vi "TCPR.vi"(0 "connection ID":refnum<k5>, 2 "错误输入（无错误）":errorcluster) -> (1 "吸液阀状态":i32, 3 "内部压力":dbl format="%.3f", 4 "外部压力":dbl format="%#.3f", 5 "连接ID输出":refnum<k5>, 6 "跟踪压力":dbl format="%.3f", 7 "错误输出":errorcluster, 8 "当前泵容量":dbl format="%.3f", 9 "排液阀状态":i32)   [LabVIEW 2014]
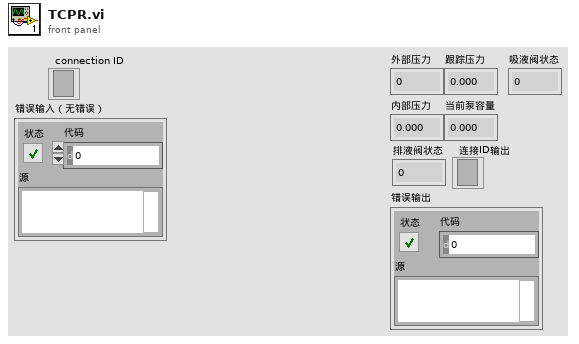
[diagram p1: front panel]
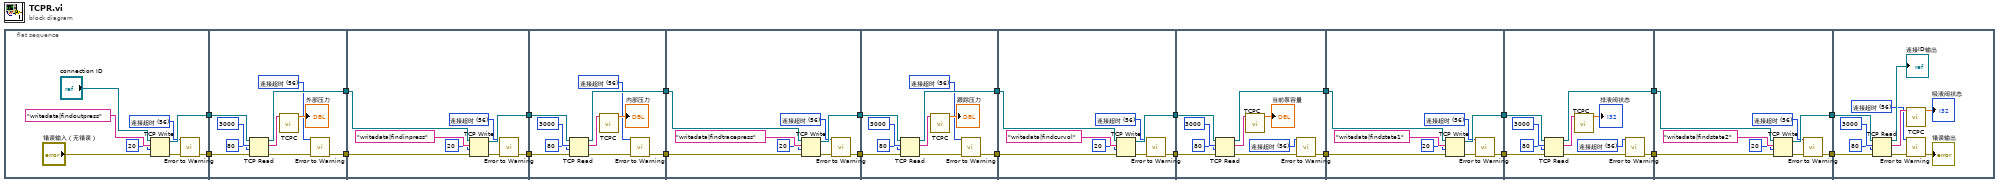
[diagram p0: block diagram]
diagram:
  n1 = flat-sequence {
    tunnel: [w24] -> w22
    tunnel: [w28] -> w21
    tunnel: w22 -> [w40]
    tunnel: w21 -> [w39]
    tunnel: [w36] -> w20
    tunnel: [w34] -> w5
    tunnel: w20 -> [w48]
    tunnel: [w46] -> w19
    tunnel: [w41] -> w6
    tunnel: w5 -> [w45]
    tunnel: w19 -> [w58]
    tunnel: [w55] -> w18
    tunnel: w6 -> [w54]
    tunnel: [w52] -> w4
    tunnel: w18 -> [w66]
    tunnel: [w64] -> w17
    tunnel: [w59] -> w7
    tunnel: w4 -> [w63]
    tunnel: w17 -> [w76]
    tunnel: [w73] -> w16
    tunnel: w7 -> [w72]
    tunnel: [w70] -> w3
    tunnel: w16 -> [w84]
    tunnel: [w82] -> w15
    tunnel: [w78] -> w8
    tunnel: w3 -> [w81]
    tunnel: w15 -> [w94]
    tunnel: [w91] -> w14
    tunnel: w8 -> [w90]
    tunnel: [w88] -> w2
    tunnel: w14 -> [w102]
    tunnel: [w100] -> w13
    tunnel: [w97] -> w9
    tunnel: w2 -> [w99]
    tunnel: w13 -> [w112]
    tunnel: [w109] -> w12
    tunnel: w9 -> [w108]
    tunnel: [w106] -> w1
    tunnel: w12 -> [w120]
    tunnel: [w118] -> w11
    tunnel: [w115] -> w10
    tunnel: w1 -> [w117]
    tunnel: w11 -> [w130]
    tunnel: w10 -> [w126]
    frame #0 {
      w23 = 56 items=["无错误", "参数错误", "内存已满", "超出区域", "文件结束", "文件已打开", "一般文件IO错误", "未找到文件", "文件权限错误", "磁盘已满", "路径副本", "打开过多文件", "未启用", "未找到资源文件", "无法添加资源", "未找到资源", "未找到图像", "图像内存错误", "画笔不存在", "配置错误类型", "配置未找到解析段", "配置解析错误", "配置内存错误", "错误外部代码格式", "错误外部代码偏移量", "外部代码不存在", "空窗口", "销毁窗口错误", "空菜单", "打印已中止", "错误打印记录", "打印驱动程序错误", "打印时窗口错误", "打印时内存错误", "打印对话框错误", "一般打印错误", "无效设备引用句柄", "设备未找到", "设备参数错误", "设备单位错误", "无法打开设备", "设备调用已中止", "一般错误", "用户已取消", "对象ID过低", "对象ID过高", "对象不在堆中", "未知的堆", "错误DefProc ID", "DefProc不在表格中", "范围外信息", "空方法", "未知信息", "不支持管理器调用", "错误地址", "连接过程中", "连接超时", "连接过程中", "不支持网络属性", "网络错误", "正在使用的地址", "系统缺少内存", "连接已中止", "连接已拒绝", "连接未建立", "连接已建立", "连接已关闭", "初始化错误（交互应用程序管理器）", "错误事件发生", "等待无约束事件发生处理程序", "事件发生队列溢出", "错误路径", "未发出信号量", "未识别类型（交互应用程序管理器）"] ("1st Error to Convert")
      n2 = TCP Write(connection ID="connection ID", data in="writedata|findoutpress" ("数据输入"), error in (no error)="错误输入（无错误）", 9:20 ("超时毫秒(25000)")) -> (connection ID out=w28:refnum<k5>, error out=w25:errorcluster)  [unwired: 1 out]
      n3 = call <vilib>:"Error to Warning.vi"("1st Error to Convert"=w23, "error in"=w25) -> ("warning out"=w24:errorcluster)  [unwired: 13 in]
    }
    frame #1 {
      w31 = 56 items=["无错误", "参数错误", "内存已满", "超出区域", "文件结束", "文件已打开", "一般文件IO错误", "未找到文件", "文件权限错误", "磁盘已满", "路径副本", "打开过多文件", "未启用", "未找到资源文件", "无法添加资源", "未找到资源", "未找到图像", "图像内存错误", "画笔不存在", "配置错误类型", "配置未找到解析段", "配置解析错误", "配置内存错误", "错误外部代码格式", "错误外部代码偏移量", "外部代码不存在", "空窗口", "销毁窗口错误", "空菜单", "打印已中止", "错误打印记录", "打印驱动程序错误", "打印时窗口错误", "打印时内存错误", "打印对话框错误", "一般打印错误", "无效设备引用句柄", "设备未找到", "设备参数错误", "设备单位错误", "无法打开设备", "设备调用已中止", "一般错误", "用户已取消", "对象ID过低", "对象ID过高", "对象不在堆中", "未知的堆", "错误DefProc ID", "DefProc不在表格中", "范围外信息", "空方法", "未知信息", "不支持管理器调用", "错误地址", "连接过程中", "连接超时", "连接过程中", "不支持网络属性", "网络错误", "正在使用的地址", "系统缺少内存", "连接已中止", "连接已拒绝", "连接未建立", "连接已建立", "连接已关闭", "初始化错误（交互应用程序管理器）", "错误事件发生", "等待无约束事件发生处理程序", "事件发生队列溢出", "错误路径", "未发出信号量", "未识别类型（交互应用程序管理器）"] ("1st Error to Convert")
      n4 = TCP Read(connection ID=w39, bytes to read=3000 ("读取的字节"), error in (no error)=w40, 9:80 ("超时毫秒(25000)")) -> (connection ID out=w36:refnum<k5>, data out=w38:string, error out=w35:errorcluster)  [unwired: 1 in]
      n5 = call "TCPC.vi"("data out"=w38) -> ("offset past number"=→"外部压力":dbl)  [unwired: 10 in]
      n6 = call <vilib>:"Error to Warning.vi"("1st Error to Convert"=w31, "error in"=w35) -> ("warning out"=w34:errorcluster)  [unwired: 13 in]
    }
    frame #2 {
      w42 = 56 items=["无错误", "参数错误", "内存已满", "超出区域", "文件结束", "文件已打开", "一般文件IO错误", "未找到文件", "文件权限错误", "磁盘已满", "路径副本", "打开过多文件", "未启用", "未找到资源文件", "无法添加资源", "未找到资源", "未找到图像", "图像内存错误", "画笔不存在", "配置错误类型", "配置未找到解析段", "配置解析错误", "配置内存错误", "错误外部代码格式", "错误外部代码偏移量", "外部代码不存在", "空窗口", "销毁窗口错误", "空菜单", "打印已中止", "错误打印记录", "打印驱动程序错误", "打印时窗口错误", "打印时内存错误", "打印对话框错误", "一般打印错误", "无效设备引用句柄", "设备未找到", "设备参数错误", "设备单位错误", "无法打开设备", "设备调用已中止", "一般错误", "用户已取消", "对象ID过低", "对象ID过高", "对象不在堆中", "未知的堆", "错误DefProc ID", "DefProc不在表格中", "范围外信息", "空方法", "未知信息", "不支持管理器调用", "错误地址", "连接过程中", "连接超时", "连接过程中", "不支持网络属性", "网络错误", "正在使用的地址", "系统缺少内存", "连接已中止", "连接已拒绝", "连接未建立", "连接已建立", "连接已关闭", "初始化错误（交互应用程序管理器）", "错误事件发生", "等待无约束事件发生处理程序", "事件发生队列溢出", "错误路径", "未发出信号量", "未识别类型（交互应用程序管理器）"] ("1st Error to Convert")
      n7 = TCP Write(connection ID=w48, data in="writedata|findinpress" ("数据输入"), error in (no error)=w45, 9:20 ("超时毫秒(25000)")) -> (connection ID out=w46:refnum<k5>, error out=w43:errorcluster)  [unwired: 1 out]
      n8 = call <vilib>:"Error to Warning.vi"("1st Error to Convert"=w42, "error in"=w43) -> ("warning out"=w41:errorcluster)  [unwired: 13 in]
    }
    frame #3 {
      w49 = 56 items=["无错误", "参数错误", "内存已满", "超出区域", "文件结束", "文件已打开", "一般文件IO错误", "未找到文件", "文件权限错误", "磁盘已满", "路径副本", "打开过多文件", "未启用", "未找到资源文件", "无法添加资源", "未找到资源", "未找到图像", "图像内存错误", "画笔不存在", "配置错误类型", "配置未找到解析段", "配置解析错误", "配置内存错误", "错误外部代码格式", "错误外部代码偏移量", "外部代码不存在", "空窗口", "销毁窗口错误", "空菜单", "打印已中止", "错误打印记录", "打印驱动程序错误", "打印时窗口错误", "打印时内存错误", "打印对话框错误", "一般打印错误", "无效设备引用句柄", "设备未找到", "设备参数错误", "设备单位错误", "无法打开设备", "设备调用已中止", "一般错误", "用户已取消", "对象ID过低", "对象ID过高", "对象不在堆中", "未知的堆", "错误DefProc ID", "DefProc不在表格中", "范围外信息", "空方法", "未知信息", "不支持管理器调用", "错误地址", "连接过程中", "连接超时", "连接过程中", "不支持网络属性", "网络错误", "正在使用的地址", "系统缺少内存", "连接已中止", "连接已拒绝", "连接未建立", "连接已建立", "连接已关闭", "初始化错误（交互应用程序管理器）", "错误事件发生", "等待无约束事件发生处理程序", "事件发生队列溢出", "错误路径", "未发出信号量", "未识别类型（交互应用程序管理器）"] ("1st Error to Convert")
      n9 = TCP Read(connection ID=w58, bytes to read=3000 ("读取的字节"), error in (no error)=w54, 9:80 ("超时毫秒(25000)")) -> (connection ID out=w55:refnum<k5>, data out=w57:string, error out=w53:errorcluster)  [unwired: 1 in]
      n10 = call "TCPC.vi"("data out"=w57) -> ("offset past number"=→"内部压力":dbl)  [unwired: 10 in]
      n11 = call <vilib>:"Error to Warning.vi"("1st Error to Convert"=w49, "error in"=w53) -> ("warning out"=w52:errorcluster)  [unwired: 13 in]
    }
    frame #4 {
      w60 = 56 items=["无错误", "参数错误", "内存已满", "超出区域", "文件结束", "文件已打开", "一般文件IO错误", "未找到文件", "文件权限错误", "磁盘已满", "路径副本", "打开过多文件", "未启用", "未找到资源文件", "无法添加资源", "未找到资源", "未找到图像", "图像内存错误", "画笔不存在", "配置错误类型", "配置未找到解析段", "配置解析错误", "配置内存错误", "错误外部代码格式", "错误外部代码偏移量", "外部代码不存在", "空窗口", "销毁窗口错误", "空菜单", "打印已中止", "错误打印记录", "打印驱动程序错误", "打印时窗口错误", "打印时内存错误", "打印对话框错误", "一般打印错误", "无效设备引用句柄", "设备未找到", "设备参数错误", "设备单位错误", "无法打开设备", "设备调用已中止", "一般错误", "用户已取消", "对象ID过低", "对象ID过高", "对象不在堆中", "未知的堆", "错误DefProc ID", "DefProc不在表格中", "范围外信息", "空方法", "未知信息", "不支持管理器调用", "错误地址", "连接过程中", "连接超时", "连接过程中", "不支持网络属性", "网络错误", "正在使用的地址", "系统缺少内存", "连接已中止", "连接已拒绝", "连接未建立", "连接已建立", "连接已关闭", "初始化错误（交互应用程序管理器）", "错误事件发生", "等待无约束事件发生处理程序", "事件发生队列溢出", "错误路径", "未发出信号量", "未识别类型（交互应用程序管理器）"] ("1st Error to Convert")
      n12 = TCP Write(connection ID=w66, data in="writedata|findtracepress" ("数据输入"), error in (no error)=w63, 9:20 ("超时毫秒(25000)")) -> (connection ID out=w64:refnum<k5>, error out=w61:errorcluster)  [unwired: 1 out]
      n13 = call <vilib>:"Error to Warning.vi"("1st Error to Convert"=w60, "error in"=w61) -> ("warning out"=w59:errorcluster)  [unwired: 13 in]
    }
    frame #5 {
      w67 = 56 items=["无错误", "参数错误", "内存已满", "超出区域", "文件结束", "文件已打开", "一般文件IO错误", "未找到文件", "文件权限错误", "磁盘已满", "路径副本", "打开过多文件", "未启用", "未找到资源文件", "无法添加资源", "未找到资源", "未找到图像", "图像内存错误", "画笔不存在", "配置错误类型", "配置未找到解析段", "配置解析错误", "配置内存错误", "错误外部代码格式", "错误外部代码偏移量", "外部代码不存在", "空窗口", "销毁窗口错误", "空菜单", "打印已中止", "错误打印记录", "打印驱动程序错误", "打印时窗口错误", "打印时内存错误", "打印对话框错误", "一般打印错误", "无效设备引用句柄", "设备未找到", "设备参数错误", "设备单位错误", "无法打开设备", "设备调用已中止", "一般错误", "用户已取消", "对象ID过低", "对象ID过高", "对象不在堆中", "未知的堆", "错误DefProc ID", "DefProc不在表格中", "范围外信息", "空方法", "未知信息", "不支持管理器调用", "错误地址", "连接过程中", "连接超时", "连接过程中", "不支持网络属性", "网络错误", "正在使用的地址", "系统缺少内存", "连接已中止", "连接已拒绝", "连接未建立", "连接已建立", "连接已关闭", "初始化错误（交互应用程序管理器）", "错误事件发生", "等待无约束事件发生处理程序", "事件发生队列溢出", "错误路径", "未发出信号量", "未识别类型（交互应用程序管理器）"] ("1st Error to Convert")
      n14 = TCP Read(connection ID=w76, bytes to read=3000 ("读取的字节"), error in (no error)=w72, 9:80 ("超时毫秒(25000)")) -> (connection ID out=w73:refnum<k5>, data out=w75:string, error out=w71:errorcluster)  [unwired: 1 in]
      n15 = call "TCPC.vi"("data out"=w75) -> ("offset past number"=→"跟踪压力":dbl)  [unwired: 10 in]
      n16 = call <vilib>:"Error to Warning.vi"("1st Error to Convert"=w67, "error in"=w71) -> ("warning out"=w70:errorcluster)  [unwired: 13 in]
    }
    frame #6 {
      w77 = 56 items=["无错误", "参数错误", "内存已满", "超出区域", "文件结束", "文件已打开", "一般文件IO错误", "未找到文件", "文件权限错误", "磁盘已满", "路径副本", "打开过多文件", "未启用", "未找到资源文件", "无法添加资源", "未找到资源", "未找到图像", "图像内存错误", "画笔不存在", "配置错误类型", "配置未找到解析段", "配置解析错误", "配置内存错误", "错误外部代码格式", "错误外部代码偏移量", "外部代码不存在", "空窗口", "销毁窗口错误", "空菜单", "打印已中止", "错误打印记录", "打印驱动程序错误", "打印时窗口错误", "打印时内存错误", "打印对话框错误", "一般打印错误", "无效设备引用句柄", "设备未找到", "设备参数错误", "设备单位错误", "无法打开设备", "设备调用已中止", "一般错误", "用户已取消", "对象ID过低", "对象ID过高", "对象不在堆中", "未知的堆", "错误DefProc ID", "DefProc不在表格中", "范围外信息", "空方法", "未知信息", "不支持管理器调用", "错误地址", "连接过程中", "连接超时", "连接过程中", "不支持网络属性", "网络错误", "正在使用的地址", "系统缺少内存", "连接已中止", "连接已拒绝", "连接未建立", "连接已建立", "连接已关闭", "初始化错误（交互应用程序管理器）", "错误事件发生", "等待无约束事件发生处理程序", "事件发生队列溢出", "错误路径", "未发出信号量", "未识别类型（交互应用程序管理器）"] ("1st Error to Convert")
      n17 = TCP Write(connection ID=w84, data in="writedata|findcurvol" ("数据输入"), error in (no error)=w81, 9:20 ("超时毫秒(25000)")) -> (connection ID out=w82:refnum<k5>, error out=w79:errorcluster)  [unwired: 1 out]
      n18 = call <vilib>:"Error to Warning.vi"("1st Error to Convert"=w77, "error in"=w79) -> ("warning out"=w78:errorcluster)  [unwired: 13 in]
    }
    frame #7 {
      w85 = 56 items=["无错误", "参数错误", "内存已满", "超出区域", "文件结束", "文件已打开", "一般文件IO错误", "未找到文件", "文件权限错误", "磁盘已满", "路径副本", "打开过多文件", "未启用", "未找到资源文件", "无法添加资源", "未找到资源", "未找到图像", "图像内存错误", "画笔不存在", "配置错误类型", "配置未找到解析段", "配置解析错误", "配置内存错误", "错误外部代码格式", "错误外部代码偏移量", "外部代码不存在", "空窗口", "销毁窗口错误", "空菜单", "打印已中止", "错误打印记录", "打印驱动程序错误", "打印时窗口错误", "打印时内存错误", "打印对话框错误", "一般打印错误", "无效设备引用句柄", "设备未找到", "设备参数错误", "设备单位错误", "无法打开设备", "设备调用已中止", "一般错误", "用户已取消", "对象ID过低", "对象ID过高", "对象不在堆中", "未知的堆", "错误DefProc ID", "DefProc不在表格中", "范围外信息", "空方法", "未知信息", "不支持管理器调用", "错误地址", "连接过程中", "连接超时", "连接过程中", "不支持网络属性", "网络错误", "正在使用的地址", "系统缺少内存", "连接已中止", "连接已拒绝", "连接未建立", "连接已建立", "连接已关闭", "初始化错误（交互应用程序管理器）", "错误事件发生", "等待无约束事件发生处理程序", "事件发生队列溢出", "错误路径", "未发出信号量", "未识别类型（交互应用程序管理器）"] ("1st Error to Convert")
      n19 = TCP Read(connection ID=w94, bytes to read=3000 ("读取的字节"), error in (no error)=w90, 9:80 ("超时毫秒(25000)")) -> (connection ID out=w91:refnum<k5>, data out=w93:string, error out=w89:errorcluster)  [unwired: 1 in]
      n20 = call "TCPC.vi"("data out"=w93) -> ("offset past number"=→"当前泵容量":dbl)  [unwired: 10 in]
      n21 = call <vilib>:"Error to Warning.vi"("1st Error to Convert"=w85, "error in"=w89) -> ("warning out"=w88:errorcluster)  [unwired: 13 in]
    }
    frame #8 {
      w96 = 56 items=["无错误", "参数错误", "内存已满", "超出区域", "文件结束", "文件已打开", "一般文件IO错误", "未找到文件", "文件权限错误", "磁盘已满", "路径副本", "打开过多文件", "未启用", "未找到资源文件", "无法添加资源", "未找到资源", "未找到图像", "图像内存错误", "画笔不存在", "配置错误类型", "配置未找到解析段", "配置解析错误", "配置内存错误", "错误外部代码格式", "错误外部代码偏移量", "外部代码不存在", "空窗口", "销毁窗口错误", "空菜单", "打印已中止", "错误打印记录", "打印驱动程序错误", "打印时窗口错误", "打印时内存错误", "打印对话框错误", "一般打印错误", "无效设备引用句柄", "设备未找到", "设备参数错误", "设备单位错误", "无法打开设备", "设备调用已中止", "一般错误", "用户已取消", "对象ID过低", "对象ID过高", "对象不在堆中", "未知的堆", "错误DefProc ID", "DefProc不在表格中", "范围外信息", "空方法", "未知信息", "不支持管理器调用", "错误地址", "连接过程中", "连接超时", "连接过程中", "不支持网络属性", "网络错误", "正在使用的地址", "系统缺少内存", "连接已中止", "连接已拒绝", "连接未建立", "连接已建立", "连接已关闭", "初始化错误（交互应用程序管理器）", "错误事件发生", "等待无约束事件发生处理程序", "事件发生队列溢出", "错误路径", "未发出信号量", "未识别类型（交互应用程序管理器）"] ("1st Error to Convert")
      n22 = TCP Write(connection ID=w102, data in="writedata|findstate1" ("数据输入"), error in (no error)=w99, 9:20 ("超时毫秒(25000)")) -> (connection ID out=w100:refnum<k5>, error out=w98:errorcluster)  [unwired: 1 out]
      n23 = call <vilib>:"Error to Warning.vi"("1st Error to Convert"=w96, "error in"=w98) -> ("warning out"=w97:errorcluster)  [unwired: 13 in]
    }
    frame #9 {
      w103 = 56 items=["无错误", "参数错误", "内存已满", "超出区域", "文件结束", "文件已打开", "一般文件IO错误", "未找到文件", "文件权限错误", "磁盘已满", "路径副本", "打开过多文件", "未启用", "未找到资源文件", "无法添加资源", "未找到资源", "未找到图像", "图像内存错误", "画笔不存在", "配置错误类型", "配置未找到解析段", "配置解析错误", "配置内存错误", "错误外部代码格式", "错误外部代码偏移量", "外部代码不存在", "空窗口", "销毁窗口错误", "空菜单", "打印已中止", "错误打印记录", "打印驱动程序错误", "打印时窗口错误", "打印时内存错误", "打印对话框错误", "一般打印错误", "无效设备引用句柄", "设备未找到", "设备参数错误", "设备单位错误", "无法打开设备", "设备调用已中止", "一般错误", "用户已取消", "对象ID过低", "对象ID过高", "对象不在堆中", "未知的堆", "错误DefProc ID", "DefProc不在表格中", "范围外信息", "空方法", "未知信息", "不支持管理器调用", "错误地址", "连接过程中", "连接超时", "连接过程中", "不支持网络属性", "网络错误", "正在使用的地址", "系统缺少内存", "连接已中止", "连接已拒绝", "连接未建立", "连接已建立", "连接已关闭", "初始化错误（交互应用程序管理器）", "错误事件发生", "等待无约束事件发生处理程序", "事件发生队列溢出", "错误路径", "未发出信号量", "未识别类型（交互应用程序管理器）"] ("1st Error to Convert")
      n24 = TCP Read(connection ID=w112, bytes to read=3000 ("读取的字节"), error in (no error)=w108, 9:80 ("超时毫秒(25000)")) -> (connection ID out=w109:refnum<k5>, data out=w111:string, error out=w107:errorcluster)  [unwired: 1 in]
      n25 = call "TCPC.vi"("data out"=w111) -> ("offset past number"=→"排液阀状态":dbl)  [unwired: 10 in]
      n26 = call <vilib>:"Error to Warning.vi"("1st Error to Convert"=w103, "error in"=w107) -> ("warning out"=w106:errorcluster)  [unwired: 13 in]
    }
    frame #10 {
      w114 = 56 items=["无错误", "参数错误", "内存已满", "超出区域", "文件结束", "文件已打开", "一般文件IO错误", "未找到文件", "文件权限错误", "磁盘已满", "路径副本", "打开过多文件", "未启用", "未找到资源文件", "无法添加资源", "未找到资源", "未找到图像", "图像内存错误", "画笔不存在", "配置错误类型", "配置未找到解析段", "配置解析错误", "配置内存错误", "错误外部代码格式", "错误外部代码偏移量", "外部代码不存在", "空窗口", "销毁窗口错误", "空菜单", "打印已中止", "错误打印记录", "打印驱动程序错误", "打印时窗口错误", "打印时内存错误", "打印对话框错误", "一般打印错误", "无效设备引用句柄", "设备未找到", "设备参数错误", "设备单位错误", "无法打开设备", "设备调用已中止", "一般错误", "用户已取消", "对象ID过低", "对象ID过高", "对象不在堆中", "未知的堆", "错误DefProc ID", "DefProc不在表格中", "范围外信息", "空方法", "未知信息", "不支持管理器调用", "错误地址", "连接过程中", "连接超时", "连接过程中", "不支持网络属性", "网络错误", "正在使用的地址", "系统缺少内存", "连接已中止", "连接已拒绝", "连接未建立", "连接已建立", "连接已关闭", "初始化错误（交互应用程序管理器）", "错误事件发生", "等待无约束事件发生处理程序", "事件发生队列溢出", "错误路径", "未发出信号量", "未识别类型（交互应用程序管理器）"] ("1st Error to Convert")
      n27 = TCP Write(connection ID=w120, data in="writedata|findstate2" ("数据输入"), error in (no error)=w117, 9:20 ("超时毫秒(25000)")) -> (connection ID out=w118:refnum<k5>, error out=w116:errorcluster)  [unwired: 1 out]
      n28 = call <vilib>:"Error to Warning.vi"("1st Error to Convert"=w114, "error in"=w116) -> ("warning out"=w115:errorcluster)  [unwired: 13 in]
    }
    frame #11 {
      w121 = 56 items=["无错误", "参数错误", "内存已满", "超出区域", "文件结束", "文件已打开", "一般文件IO错误", "未找到文件", "文件权限错误", "磁盘已满", "路径副本", "打开过多文件", "未启用", "未找到资源文件", "无法添加资源", "未找到资源", "未找到图像", "图像内存错误", "画笔不存在", "配置错误类型", "配置未找到解析段", "配置解析错误", "配置内存错误", "错误外部代码格式", "错误外部代码偏移量", "外部代码不存在", "空窗口", "销毁窗口错误", "空菜单", "打印已中止", "错误打印记录", "打印驱动程序错误", "打印时窗口错误", "打印时内存错误", "打印对话框错误", "一般打印错误", "无效设备引用句柄", "设备未找到", "设备参数错误", "设备单位错误", "无法打开设备", "设备调用已中止", "一般错误", "用户已取消", "对象ID过低", "对象ID过高", "对象不在堆中", "未知的堆", "错误DefProc ID", "DefProc不在表格中", "范围外信息", "空方法", "未知信息", "不支持管理器调用", "错误地址", "连接过程中", "连接超时", "连接过程中", "不支持网络属性", "网络错误", "正在使用的地址", "系统缺少内存", "连接已中止", "连接已拒绝", "连接未建立", "连接已建立", "连接已关闭", "初始化错误（交互应用程序管理器）", "错误事件发生", "等待无约束事件发生处理程序", "事件发生队列溢出", "错误路径", "未发出信号量", "未识别类型（交互应用程序管理器）"] ("1st Error to Convert")
      n29 = TCP Read(connection ID=w130, bytes to read=3000 ("读取的字节"), error in (no error)=w126, 9:80 ("超时毫秒(25000)")) -> (connection ID out=→"连接ID输出":refnum<k5>, data out=w129:string, error out=w125:errorcluster)  [unwired: 1 in]
      n30 = call "TCPC.vi"("data out"=w129) -> ("offset past number"=→"吸液阀状态":dbl)  [unwired: 10 in]
      n31 = call <vilib>:"Error to Warning.vi"("1st Error to Convert"=w121, "error in"=w125) -> ("warning out"=→"错误输出":errorcluster)  [unwired: 13 in]
    }
  }
